vi "osc2.vi"() -> ()   [LabVIEW 2016]
uses:
  <instrlib>/Tektronix TDS 200 1000 2000 Series/Public/Data/Read (Multiple Waveforms).vi
  <instrlib>/Tektronix TDS 200 1000 2000 Series/Tektronix TDS 200 1000 2000 Series.lvlib
panel:
  out "Waveform Data":waveform(dbl)[](graph)
  in  "VISA resource name":refnum<visa-resource-name>
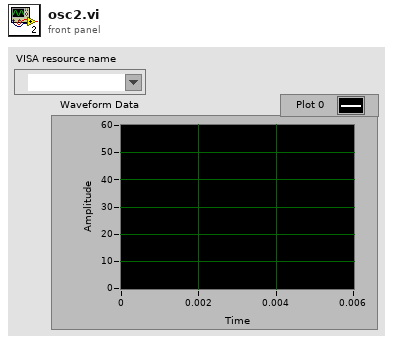
[diagram p1: front panel]
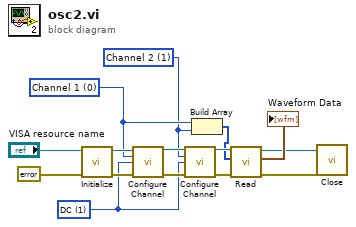
[diagram p0: block diagram]
diagram:
  w9 = 1 items=["AC", "DC", "Ground"] ("Vertical Coupling (1: DC)")
  w5 = 1 items=["Channel 1", "Channel 2", "Channel 3", "Channel 4", "Math", "Reference A", "Reference B", "Reference C", "Reference D"] ("Channel (0: Channel 1)")
  w6 = 0 items=["Channel 1", "Channel 2", "Channel 3", "Channel 4", "Math", "Reference A", "Reference B", "Reference C", "Reference D"] ("Channel (0: Channel 1)")
  n1 = call <instrlib>:"Initialize.vi"("error in (no error)"=errorcluster {"status"=FALSE, "code"=0, "source"=""}, "VISA resource name"="VISA resource name") -> ("error out"=w11:errorcluster, "VISA resource name out"=w13:refnum<visa-resource-name>)  [unwired: 8 in]
  n2 = call <instrlib>:"Configure Channel.vi"("VISA resource name"=w13, "Channel (0: Channel 1)"=w6, "Vertical Coupling (1: DC)"=w9, "error in (no error)"=w11) -> ("VISA resource name out"=w12:refnum<visa-resource-name>, "error out"=w10:errorcluster)  [unwired: 10 in]
  n3 = call <instrlib>:"Configure Channel.vi"("VISA resource name"=w12, "Channel (0: Channel 1)"=w5, "Vertical Coupling (1: DC)"=w9, "error in (no error)"=w10) -> ("VISA resource name out"=w7:refnum<visa-resource-name>, "error out"=w8:errorcluster)  [unwired: 10 in]
  n4 = Build Array(w6, w5) -> (w4:i32[])
  n5 = call-poly <instrlib>:"Read.vi"("error in (no error)"=w8, "Channels"=w4, "VISA resource name"=w7) -> ("error out"=w2:errorcluster, "Waveform Data"=→"Waveform Data":waveform(dbl)[], "VISA resource name out"=w1:refnum<visa-resource-name>)  [unwired: 6 in]
  n6 = call <instrlib>:"Close.vi"("error in (no error)"=w2, "VISA resource name"=w1) -> ()  [unwired: 9 in, 1 out]
